vi "GenerateError.vi"(8 "error in":errorcluster, 11 "error_code":T1 items=["none"=0, "busy"=65536, "error"=131072, "parameter"=262144, "locked"=524288, "sync"=1048576, "connection"=2097152, "internal"=4194304, "end_of_data"=8388608]) -> (0 "error out":errorcluster)   [LabVIEW 2020]
uses:
  DEFINITIONS/DEF_T_error_enum.ctl
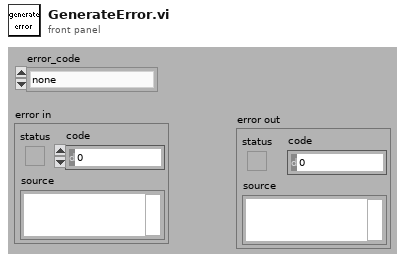
[diagram p1: front panel]
types:
  T1 = typedef "DEF_T_error_enum.ctl" = u32
  T2 = typedef "LVStringsAndValuesArrayTypeDef_U32.ctl" = cluster{"String":string, "Value":u32}[]
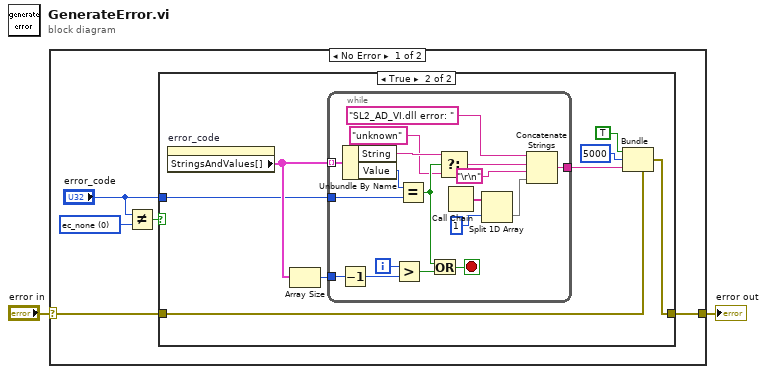
[diagram p0: block diagram]
diagram:
  n1 = case shown="No Error" "error in" {
    selector: "error in" -> [w3 w35]
    tunnel: [w4 w35] -> w2
    frame No Error {
      w7 = T1 0 items=["ec_none"=0, "ec_busy"=65536, "ec_error"=131072, "ec_parameter"=262144, "ec_locked"=524288, "ec_sync"=1048576, "ec_nonnection"=2097152, "ec_internal"=4194304, "ec_end_of_data"=8388608] ("error_code")
      n2 = Not Equal?(x="error_code", y=w7) -> (x != y?=w5:bool)
      n3 = case shown="True" w5 {
        tunnel: w3 -> [w8 w16]
        tunnel: "error_code" -> [_ w11]
        tunnel: [w8 w9] -> w4
        frame False {
        }
        frame True {
          n4 = property on="error_code" class="Ring (strict)"() -> ("StringsAndValues[]"=w13:T2)  [unwired: 2 in, 2 out]
          n5 = Array Size(array=w13) -> (size(s)=w12:i32)
          n6 = while {
            tunnel: w13 -> [w34] mode=indexing
            tunnel: w12 -> [w30]
            tunnel: w11 -> [w32]
            tunnel: [w20] -> w10
            i -> [w31]
            stop <- w27 stop-if-true
            n7 = Decrement(x=w30) -> (x-1=w29:i32)
            n8 = Unbundle By Name(w34) -> ("String"=w25:string, "Value"=w33:u32)
            n9 = Greater?(x=w31, y=w29) -> (0:w28:bool)
            n10 = Equal?(x=w33, y=w32) -> (x = y?=w26:bool)
            n11 = Or(x=w26, y=w28) -> (x .or. y?=w27:bool)
            n12 = Select(t=w25, s=w26, f="unknown") -> (s? t:f=w22:string)
            n13 = Call Chain() -> (call chain=w19:string[])
            n14 = Split 1D Array(array=w19, index=1) -> (second subarray=w17:string[])  [unwired: 1 out]
            n15 = Concatenate Strings("SL2_AD_VI.dll error: ", w22, "\r\n", w17) -> (w20:string)
          }
          n16 = Bundle(cluster=w16, "status"=TRUE, "code"=5000, "source"=w10) -> (w9:errorcluster)
        }
      }
    }
    frame Error {
    }
  }
  "error out" <- w2
